vi "Dashboard Main.vi"() -> ()   [LabVIEW 2013]
uses:
  2014 Target Detection/TargetType.ctl
  <vilib>/event_ctls.llb/eventvkey.ctl
  <vilib>/Rock Robotics/WPI/Dashboard/WPI_DashboardLogging Global.vi
  <vilib>/Utility/config.llb/Write Key (String).vi
  <vilib>/Utility/config.llb/Write Key (I32).vi
  <vilib>/Utility/config.llb/NI_LVConfig.lvlib
panel:
  out "Image Message":string="Timeout in Camera Communications"
  in  "Rec Mode":enum32{"Stop", "Record", "Playback"}(radio)
  in  "Dashboard Tab":T1(tab)=enum."Auto"
  in  "Camera Settings":T2={"Frame Rate"=30, "Compression"=30, "Size"=1} {"Frame Rate" scale=1.0..30.0; "Size" items=["640x480", "320x240", "160x120"]}
  out "MotorSliders R":cluster{"MotorSlide1":dbl, "MotorSlide2":dbl}={"MotorSlide1"=0.0, "MotorSlide2"=-6.200012400024799e-05} {"MotorSlide2" scale=-1.0..1.0 scale format="%#_2e"; "MotorSlide1" scale=-1.0..1.0 scale format="%#_2e"}
  out "MotorChart R":cluster{"Numeric":dbl, "Numeric":dbl}(graph)={"Numeric"=0.0, "Numeric"=-6.200012400024799e-05}
  out "MotorSliders L":T3={"MotorSlide1"=0.0, "MotorSlide2"=-6.200012400024799e-05, "MotorSlide4 2"=12.519999504089355} {"MotorSlide4 2" scale=0.0..14.0 scale format="%#_2e"; "MotorSlide2" scale=-1.0..1.0 scale format="%#_2e"; "MotorSlide1" scale=-1.0..1.0 scale format="%#_2e"}
  out "MotorChart L":T4(graph)={"Numeric"=0.0, "Numeric"=-6.200012400024799e-05, "Battery"=12.5199995}
  out "JS1 Z":dbl(slide)=-1.0 scale=-1.0..1.0 scale format="%#_2e"
  out "Joystick 1":cluster{"X":dbl, "Y":dbl}[](graph)=[{"X"=-0.007874015748031496, "Y"=0.0}]
  out "JS Buttons 1":T5
  out "JS2 Z":dbl(slide) scale=-1.0..1.0 scale format="%#_2e"
  out "Joystick 2":cluster{"X":dbl, "Y":dbl}[](graph)
  out "JS Buttons 2":T5
  out "Mode":T6(ring)
  out "Camera IP":string="10.43.81.11"
  in  "DB Camera Config":bool
  out "fps":dbl=32.432432432432435 format="%#.1g"
  out "Mbps":dbl=3.953641040546432 format="%#.1g"
  out "Mbps 2":bool
  out "LED 1":bool
  in  "Slider 1":dbl(slide) scale=0.0..100.0
  out "Distances":T8(array[cluster])=[{"Distance (ft)"=9.467013752624329, "Target Center (-1 to 1)"={"X"=0.2125, "Y"=-0.19583333333333333}, "Left"=FALSE, "State"=enum."Hot"}]
  in  "Color Components":T9={"Hue"={96.67088317871094, 128.67088317871094}, "Sat"={183.00372314453125, 255.0}, "Val"={112.86207389831543, 166.60627937316895}} {"Val" scale=0.0..255.0; "Sat" scale=0.0..255.0; "Hue" scale=0.0..255.0 scale format="%#_3g"}
  in  "Checkbox 2":bool
  in  "Checkbox 1":bool
  in  "Test Slider":dbl(slide) scale=0.0..100.0 scale format="%#_3g"
  in  "On/Off":bool caption="Solenoid"
  in  "Test Name":u16(ring) items=["Select the test to run...", "Example Test", "-------------------------------", "List of tests is built in robot code.", "Replace with your own automated tests."]
  in  "Test Tree":string(tree)
  in  "Motor":cluster{"Value":dbl, "Enable":bool} {"Value" scale=-1.0..1.0 scale format="%#_3g"}
  out "Progress":T10 {"Test Progress" scale=0.0..100.0}
  in  "Rev/Fwd":cluster{"Forward":bool, "Reverse":bool}
  in  "Test Ring":u16(ring) items=["Auto", "Fixed indoor", "Fixed outdoor 1", "Fixed outdoor 2", "Fixed fluorescent 1", "Fixed fluorescent 2", "Hold current"]
  in  "Listbox":i32(listbox)
  out "Tree":string(tree)
  out "Camera Image":T11(plugin-control)
  in  "Enable":bool=TRUE
  # "Left"
  # "Front"
  # "Right"
  # "Battery"
  # "Customize by placing controls and indicators here and name to\nmatch Dashboard Variables on robot."
  # "This tab is a great place for autonomous settings and validation.\nCustomize by placing controls and indicators here and name to\nmatch Dashboard Variables on robot."
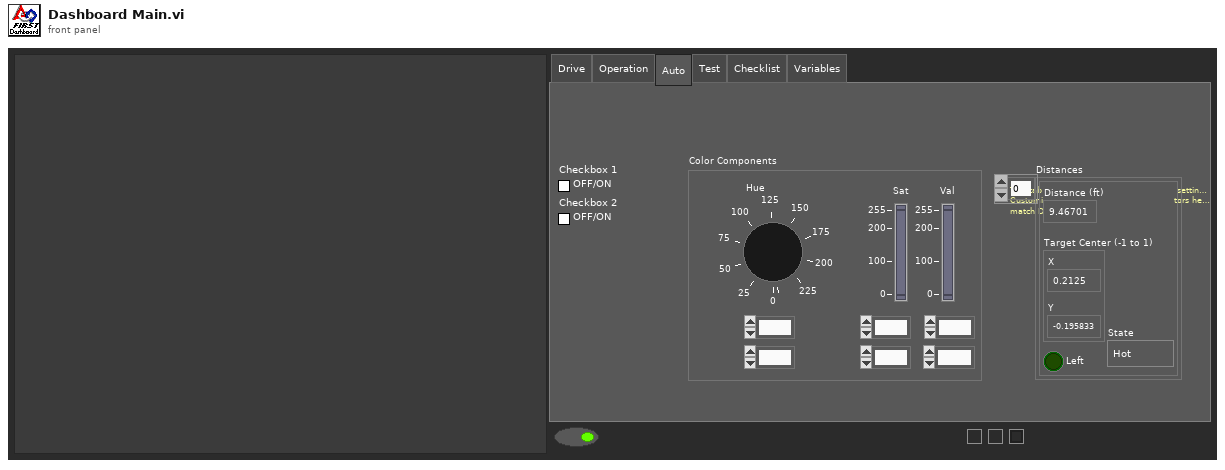
[diagram p1: front panel]
types:
  T1 = enum32{"Drive", "Operation", "Auto", "Test", "Checklist", "Variables"}
  T2 = cluster{"Frame Rate":i32, "Compression":i32, "Size":u16}
  T3 = cluster{"MotorSlide1":dbl, "MotorSlide2":dbl, "MotorSlide4 2":dbl}
  T4 = cluster{"Numeric":dbl, "Numeric":dbl, "Battery":sgl}
  T5 = cluster{bool, bool, bool, bool, bool, bool, bool, bool, bool, bool, bool, bool}
  T6 = enum8{"Tele-Op Disabled", "Tele-Op Enabled", "Auto Disabled", "Auto Enabled", "Test Disabled", "Test Enabled", ""}
  T7 = typedef "TargetType.ctl" = enum16{"Not Hot", "Hot"}
  T8 = cluster{"Distance (ft)":dbl, "Target Center (-1 to 1)":cluster{"X":dbl, "Y":dbl}, "Left":bool, "State":T7}[]
  T9 = cluster{"Hue":cluster{dbl, dbl}, "Sat":cluster{dbl, dbl}, "Val":cluster{dbl, dbl}}
  T10 = cluster{"Test Progress":u8, "Test Progress Text":string}
  T11 = typedef "IMAQ Image.ctl" = refnum<image>
  T12 = typedef "Image Type" = u32
  T13 = cluster{cluster{dbl, dbl}, cluster{dbl, dbl}, cluster{dbl, dbl}}
  T14 = cluster{"Digital Inputs":bool[], "Digital Outputs":bool[]}
  T15 = cluster{"Competition mode":bool, "Robot Link":bool, "Autonomous":bool, "Enabled":bool, "E-Stop":bool, "Simulated":bool, "TestMode":bool, "Docked Window":bool}
  T16 = cluster{"Boolean Array[0]":bool, "Boolean Array[1]":bool, "Boolean Array[2]":bool, "Boolean Array[3]":bool, "Boolean Array[4]":bool, "Boolean Array[5]":bool, "Boolean Array[6]":bool, "Boolean Array[7]":bool, "Boolean Array[8]":bool, "Boolean Array[9]":bool, "Boolean Array[10]":bool, "Boolean Array[11]":bool}
  T17 = typedef "NI_LVConfig.lvlib/Config Data RefNum.ctl" = refnum<k1>
  T18 = typedef "eventvkey.ctl" = enum16{"ASCII", "Enter", "Return", "Shift", "Ctrl", "Alt", "Cmd", "Opt", "Caps", "NumLock", "Clear", "Break", "Up", "Down", "Left", "Right", "Insert", "Delete", "Home", "End", "PageUp", "PageDown", "Escape", "Help", "Pause", "ScrollLock", "F1", "F2", "F3", "F4", "F5", "F6", "F7", "F8", "F9", "F10", "F11", "F12", "F13", "F14", "F15", "F16", "F17", "F18", "F19", "F20", "F21", "F22", "F23", "F24", "Play", "VolumeUp", "VolumeDown", "Mute", "Two Byte Char"}
  T19 = cluster{"Image Size":bool, "Image Type":bool, "Pixel Value":bool, "ROI Information":bool, "Zoom Factor":bool}
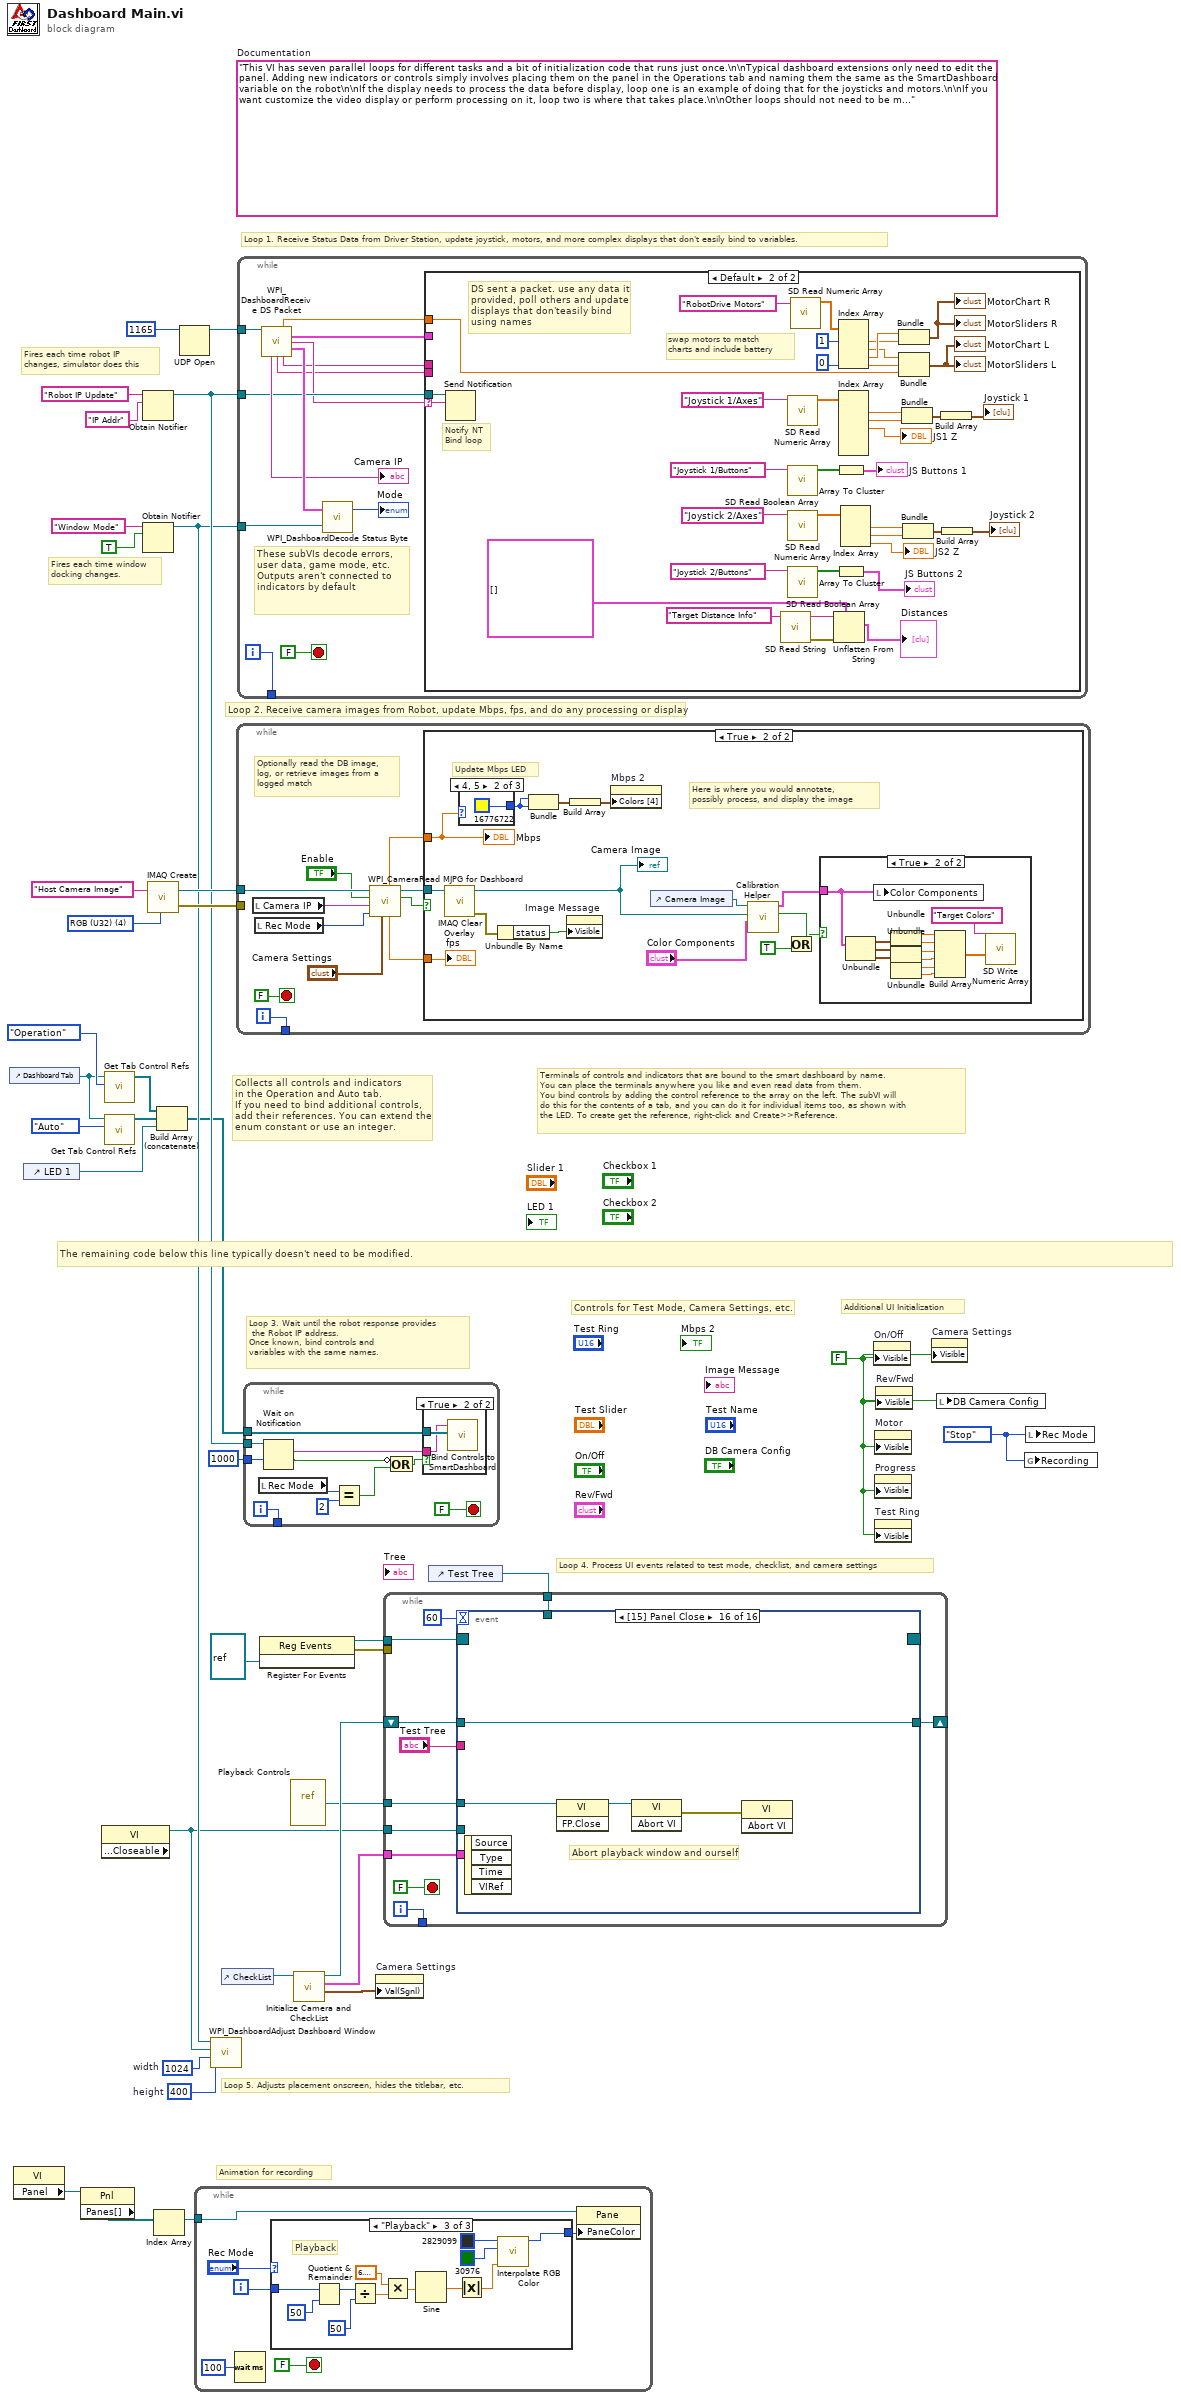
[diagram p0: block diagram]
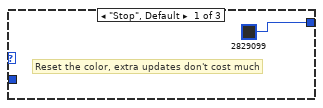
[diagram p2: hidden frame]
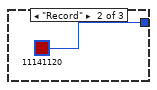
[diagram p3: hidden frame]
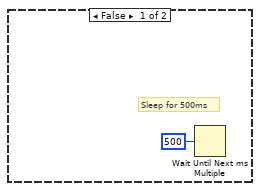
[diagram p5: hidden frame]
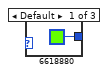
[diagram p7: hidden frame]
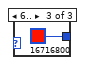
[diagram p8: hidden frame]
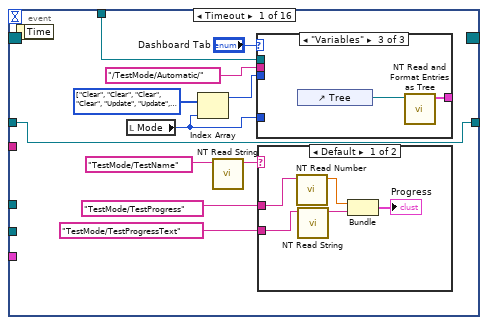
[diagram p9: hidden frame]
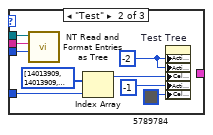
[diagram p11: hidden frame]
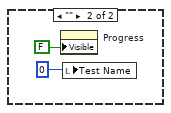
[diagram p12: hidden frame]
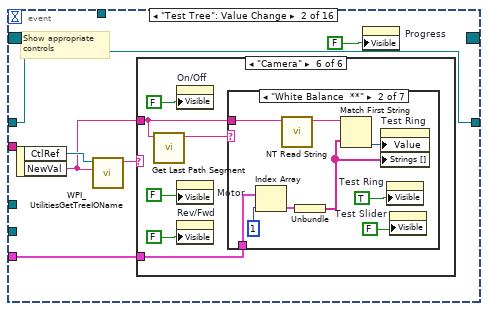
[diagram p13: hidden frame]
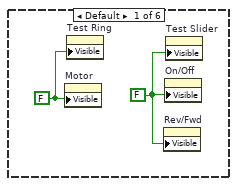
[diagram p14: hidden frame]
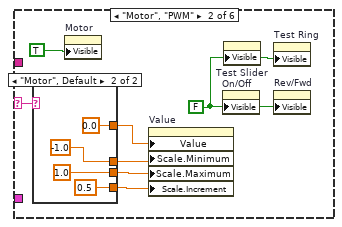
[diagram p15: hidden frame]
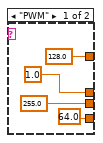
[diagram p16: hidden frame]
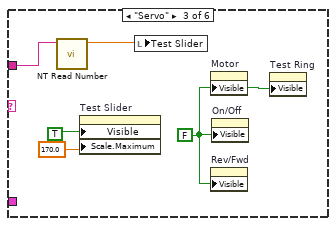
[diagram p17: hidden frame]
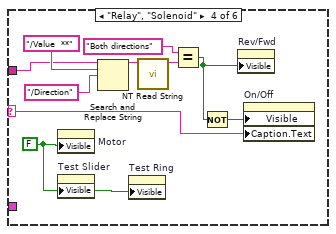
[diagram p18: hidden frame]
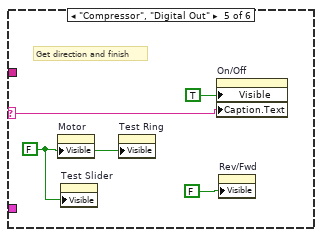
[diagram p19: hidden frame]
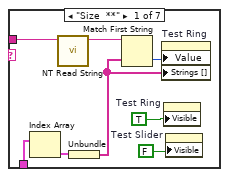
[diagram p20: hidden frame]
diagram:
  w8 = enum32{"Stop", "Record", "Playback"}."Stop" ("Rec Mode")
  w11 = 400  # height
  w12 = 1024  # width
  w25 = FALSE ("Visible")
  (unwired) "This VI has seven parallel loops for different tasks and a bit of initialization code that runs just once.\n\nTypical dashboard extensions only need to edit the panel. Adding new indicators or controls simply involves placing them on the panel in the Operations tab and naming them the same as the SmartDashboard variable on the robot\n\nIf the display needs to process the data before display, loop one is an example of doing that for the joysticks and motors.\n\nIf you want customize the video display or perform processing on it, loop two is where that takes place.\n\nOther loops should not need to be modified. They are pretty standard, and document the task they perform."  # Documentation
  w35 = T12 4 items=["Grayscale (U8)", "Grayscale (I16)", "Grayscale (SGL)", "Complex (CSG)", "RGB (U32)", "HSL (U32)", "RGB (U64)"] ("Image Type")
  # "Controls for Test Mode, Camera Settings, etc."
  # "Additional UI Initialization"
  # "Animation for recording"
  # "Fires each time robot IP\nchanges, simulator does this"
  # "Fires each time window\ndocking changes."
  # "Collects all controls and indicators\nin the Operation and Auto tab.\nIf you need to bind additional controls,\nadd their references. You can extend the\nenum constant or use an integer."
  # "The remaining code below this line typically doesn't need to be modified."
  # "Loop 4. Process UI events related to test mode, checklist, and camera settings"
  # "Terminals of controls and indicators that are bound to the smart dashboard by name.\nYou can place the terminals anywhere you like and even read data from them.\nYou bind controls by adding the control reference to the array on the left. The subVI will\ndo this for the contents of a tab, and you can do it for individual items too, as shown with\nthe LED. To create get the reference, right-click and Create>>Reference."
  # "Loop 3. Wait until the robot response provides\n the Robot IP address.\nOnce known, bind controls and\nvariables with the same names."
  # "Loop 5. Adjusts placement onscreen, hides the titlebar, etc."
  # "Loop 1. Receive Status Data from Driver Station, update joystick, motors, and more complex displays that don't easily bind to variables."
  # "Loop 2. Receive camera images from Robot, update Mbps, fps, and do any processing or display"
  n1 = control-ref of="Dashboard Tab"() -> (w6:refnum<vi>)
  n2 = property class="VI"() -> ("Panel"=w19:refnum<vi>)  [unwired: 2 in, 2 out]
  n3 = control-ref of="LED 1"() -> (w1:refnum<vi>)
  n4 = property class="Pnl"(reference=w19) -> ("Panes[]"=w20:refnum<vi>[])  [unwired: 1 in, 2 out]
  n5 = property class="VI" props=["Front Panel.Closeable"]() -> (reference out=w7:refnum<vi>)  [unwired: 2 in, 2 out]
  n6 = call <vilib>:"Get Tab Control Refs.vi"("Page Index"=T1."Operation" ("Dashboard Tab"), "TabControl in"=w6) -> ("ControlsOnPage"=w4:refnum<vi>[])  [unwired: 9 in]
  n7 = call <vilib>:"Get Tab Control Refs.vi"("Page Index"=T1."Auto" ("Dashboard Tab"), "TabControl in"=w6) -> ("ControlsOnPage"=w5:refnum<vi>[])  [unwired: 9 in]
  n8 = Obtain Notifier(name (unnamed)="Robot IP Update", notification data type="IP Addr" ("name (unnamed)")) -> (notifier out=w29:refnum<notifier>)  [unwired: 2 in, 2 out]
  n9 = Obtain Notifier(name (unnamed)="Window Mode", notification data type=TRUE) -> (notifier out=w10:refnum<notifier>)  [unwired: 2 in, 2 out]
  n10 = call "IMAQ Create"("Image Name"="Host Camera Image", "Image Type"=w35) -> ("New Image"=w33:T11, "error out"=w32:errorcluster)  [unwired: 2 in, 1 out]
  n11 = Index Array(array=w20) -> (element=w18:refnum<vi>)  [unwired: 1 in]
  n12 = Build Array (concatenate)(w4, w5, w1) -> (w3:refnum<vi>[])
  n13 = UDP Open(11:u16 1165 ("port")) -> (port=w36:refnum<k16>)  [unwired: 2 in, 4 out]
  n14 = while {
    tunnel: w18 -> [w39]
    i -> [w42]
    stop <- FALSE stop-if-true
    n15 = Wait (ms)(milliseconds to wait=u32 100) -> ()  [unwired: 1 out]
    n16 = case shown="\"Playback\"" "Rec Mode" {
      tunnel: w42 -> [_ _ w57]
      tunnel: [u32 2829099 ("Base Color") u32 11141120 ("Target Color") w46] -> w38
      frame "Stop", Default {
        # "Reset the color, extra updates don't cost much"
      }
      frame "Record" {
      }
      frame "Playback" {
        # "Playback"
        n17 = Quotient & Remainder(x=w57, y=u32 50 ("milliseconds to wait")) -> (x-y*floor(x/y)=w53:u32)  [unwired: 1 out]
        n18 = Divide(x=w53, y=u32 50 ("milliseconds to wait")) -> (x/y=w50:dbl)
        n19 = Multiply(x=6.283185307179586, y=w50) -> (x*y=w55:dbl)
        n20 = Sine(x=w55) -> (sin(x)=w54:dbl)
        n21 = Absolute Value(x=w54) -> (abs(x)=w47:dbl)
        n22 = call "Interpolate RGB Color.vi"("Proportion"=w47, "Target Color"=u32 30976, "Base Color"=u32 2829099) -> ("Result Color"=w46:u32)  [unwired: 8 in]
      }
    }
    n23 = property class="Pane"(reference=w39, "PaneColor"=w38) -> ()  [unwired: 1 in, 2 out]
  }
  n24 = call <vilib>:"WPI_DashboardAdjust Dashboard Window.vi"("height"=w11, "width"=w12, "reference in"=w7, "Notifier in"=w10) -> ()  [unwired: 8 in]
  n25 = control-ref of="CheckList"() -> (w9:refnum<vi>)
  n26 = while {
    tunnel: w33 -> [w66]
    tunnel: w32 -> [_]
    tunnel: [w67] -> _
    i -> [w67]
    stop <- FALSE stop-if-true
    # "Optionally read the DB image,\nlog, or retrieve images from a\nlogged match"
    n27 = local read "Camera IP"() -> (w59:string)
    n28 = local read "Rec Mode"() -> (w58:enum32{"Stop", "Record", "Playback"})
    n29 = call <vilib>:"WPI_CameraRead MJPG for Dashboard.vi"("Camera Settings"="Camera Settings", "Rec Mode"=w58, "Camera IP"=w59, "Enable"="Enable", "Refnum in"=w66) -> ("Active"=w63:bool, "Refnum out"=w65:T11, "FPS"=w62:dbl, "Bandwidth (Mbps)"=w61:dbl)  [unwired: 3 in]
    n30 = case shown="True" w63 {
      tunnel: w65 -> [_ w79]
      tunnel: w61 -> [_ w78]
      tunnel: w62 -> [_ w77]
      frame False {
        # "Sleep for 500ms"
        n31 = Wait Until Next ms Multiple(millisecond multiple=u32 500) -> ()  [unwired: 1 out]
      }
      frame True {
        # "Here is where you would annotate,\npossibly process, and display the image"
        # "Update Mbps LED"
        n32 = call "IMAQ Clear Overlay"("Image"=w79) -> ("error out"=w83:errorcluster, "Image Out"=w76:T11)  [unwired: 2 in, 7 out]
        "Camera Image" <- w76
        n33 = case shown="4, 5" w78 {
          tunnel: [u32 6618880 ("Color Box") u32 16776722 ("Color Box") u32 16716800 ("Color Box")] -> w80
          frame Default {
          }
          frame 4, 5 {
          }
          frame 6.. {
          }
        }
        n34 = Unbundle By Name(w83) -> ("status"=w84:bool)
        n35 = Bundle("Color Box"=w80, "Color Box"=w80) -> (w82:cluster{"Color Box":u32, "Color Box":u32})  [unwired: 1 out]
        n36 = property on="Image Message" class="Str"("Visible"=w84) -> ()  [unwired: 2 in, 2 out]
        n37 = Build Array(w82) -> (w81:cluster{"Color Box":u32, "Color Box":u32}[])
        n38 = property on="Mbps 2" class="Bool (strict)"("Colors [4]"=w81) -> ()  [unwired: 2 in, 2 out]
        n39 = control-ref of="Camera Image"() -> (w75:refnum<vi>)
        n40 = call "Calibration Helper.vi"("Color Components"="Color Components", "Image"=w76, "Image Ctl Refnum"=w75) -> ("Changed"=w72:bool, "output color"=w73:T13)  [unwired: 7 in]
        n41 = Or(x=w72, y=TRUE) -> (x .or. y?=w70:bool)
        n42 = case shown="True" w70 {
          tunnel: w73 -> [_ w96]
          frame False {
          }
          frame True {
            n43 = Unbundle(w96) -> (w95:cluster{dbl, dbl}, w94:cluster{dbl, dbl}, w93:cluster{dbl, dbl})
            n44 = local write "Color Components"(w96) -> ()
            n45 = Unbundle(w95) -> (w92:dbl, w91:dbl)
            n46 = Unbundle(w94) -> (w90:dbl, w89:dbl)
            n47 = Unbundle(w93) -> (w88:dbl, w87:dbl)
            n48 = Build Array(w92, w91, w90, w89, w88, w87) -> (w86:dbl[])
            n49 = call <vilib>:"SD Write Numeric Array.vi"("Numeric Array"=w86, "Name"="Target Colors") -> ()  [unwired: 8 in, 2 out]
          }
        }
        "Mbps" <- w78
        "fps" <- w77
      }
    }
  }
  n50 = while {
    tunnel: w36 -> [w110]
    tunnel: w29 -> [w105]
    tunnel: w10 -> [w109]
    tunnel: [w106] -> _
    i -> [w106]
    stop <- FALSE stop-if-true
    # "These subVIs decode errors, user data, game mode, etc.\nOutputs aren't connected to indicators by default"
    n51 = call <vilib>:"WPI_DashboardReceive DS Packet.vi"("Recv Socket"=w110) -> ("Battery"=w100:sgl, "Driver Station"=w101:T14, "Robot IP Address"=w104:string, "Status"=w111:T15, "Camera IP Address"=→"Camera IP":string, "Low Priority User Data"=w103:string, "High Priority User Data"=w102:string)  [unwired: 1 in, 7 out]
    n52 = call <vilib>:"WPI_DashboardDecode Status Byte.vi"("Window Mode Notifier"=w109, "Status"=w111) -> ("Mode"=→"Mode":T6)  [unwired: 1 out]
    n53 = case shown="Default" w104 {
      selector: w104 -> [_ w128]
      tunnel: w105 -> [_ w129]
      tunnel: w103 -> [_ _]
      tunnel: w102 -> [_ _]
      tunnel: w101 -> [_ _]
      tunnel: w100 -> [_ w127]
      frame "0.0.0.0" {
        # "DS not sending packets, or no robot exists yet.\nDon't poll the variables"
      }
      frame Default {
        # "Notify NT\nBind loop"
        # "DS sent a packet. use any data it\nprovided, poll others and update\ndisplays that don'teasily bind\nusing names"
        # "swap motors to match\ncharts and include battery"
        n54 = Send Notification(notification=w128, notifier=w129) -> ()  [unwired: 1 in, 2 out]
        n55 = call <vilib>:"SD Read String.vi"("Name"="Target Distance Info") -> ("error out"=w117:errorcluster, "String"=w116:string)  [unwired: 8 in, 1 out]
        n56 = call <vilib>:"SD Read Numeric Array.vi"("Name"="Joystick 1/Axes") -> ("Numeric Array"=w145:dbl[])  [unwired: 8 in, 2 out]
        n57 = call <vilib>:"SD Read Boolean Array.vi"("Name"="Joystick 1/Buttons") -> ("Boolean Array"=w147:bool[])  [unwired: 8 in, 2 out]
        n58 = call <vilib>:"SD Read Numeric Array.vi"("Name"="Joystick 2/Axes") -> ("Numeric Array"=w139:dbl[])  [unwired: 8 in, 2 out]
        n59 = call <vilib>:"SD Read Boolean Array.vi"("Name"="Joystick 2/Buttons") -> ("Boolean Array"=w138:bool[])  [unwired: 8 in, 2 out]
        n60 = call <vilib>:"SD Read Numeric Array.vi"("Name"="RobotDrive Motors") -> ("Numeric Array"=w126:dbl[])  [unwired: 8 in, 2 out]
        n61 = Unflatten From String(type=T8 [] ("Distances"), binary string=w116, error in (no error)=w117) -> (value=→"Distances":T8)  [unwired: 2 in, 2 out]
        n62 = Array To Cluster(array=w147) -> (cluster=→"JS Buttons 1":T16)
        n63 = Array To Cluster(array=w138) -> (cluster=→"JS Buttons 2":T16)
        n64 = Index Array(array=w126, index #1=1, index #4=0) -> (element #1=w122:dbl, element #2=w121:dbl, element #3=w123:dbl, element #4=w118:dbl)  [unwired: 2 in]
        n65 = Index Array(array=w145) -> (element #1=w142:dbl, element #2=w143:dbl, element #3=→"JS1 Z":dbl)  [unwired: 6 in, 3 out]
        n66 = Index Array(array=w139) -> (element #1=w134:dbl, element #2=w133:dbl, element #3=→"JS2 Z":dbl)  [unwired: 3 in]
        n67 = Bundle("Numeric"=w123, "Numeric"=w122) -> (→"MotorChart R" →"MotorSliders R":cluster{"Numeric":dbl, "Numeric":dbl})  [unwired: 1 in]
        n68 = Bundle("Numeric"=w121, "Numeric"=w118, "Battery"=w127) -> (→"MotorChart L" →"MotorSliders L":T4)  [unwired: 1 in]
        n69 = Bundle("Numeric"=w142, "Numeric"=w143) -> (w141:cluster{"Numeric":dbl, "Numeric":dbl})  [unwired: 1 in]
        n70 = Bundle("Numeric"=w134, "Numeric"=w133) -> (w135:cluster{"Numeric":dbl, "Numeric":dbl})  [unwired: 1 in]
        n71 = Build Array(w141) -> (→"Joystick 1":cluster{"Numeric":dbl, "Numeric":dbl}[])
        n72 = Build Array(w135) -> (→"Joystick 2":cluster{"Numeric":dbl, "Numeric":dbl}[])
      }
    }
  }
  n73 = while {
    tunnel: w3 -> [w161]
    tunnel: w29 -> [w159]
    tunnel: [w157] -> _
    tunnel: u32 1000 ("milliseconds to wait") -> [w156]
    i -> [w157]
    stop <- FALSE stop-if-true
    n74 = local read "Rec Mode"() -> (w152:enum32{"Stop", "Record", "Playback"})
    n75 = Wait on Notification(notifier=w159, timeout in ms (-1)=w156) -> (notification=w158:string, timed out?=w154:bool)  [unwired: 2 in, 2 out]
    n76 = Equal?(x=w152, y=u16 2 ("Rec Mode")) -> (x = y?=w153:bool)
    n77 = Compound Arithmetic op=OR(invert w154, w153) -> (w155:bool)
    n78 = case shown="True" w155 {
      tunnel: w161 -> [_ w163]
      tunnel: w158 -> [_ w162]
      frame False {
      }
      frame True {
        n79 = call <vilib>:"Bind Controls to SmartDashboard.vi"("Bound Control Refs"=w163, "Server IP Address"=w162) -> ()  [unwired: 10 in]
      }
    }
  }
  n80 = register-events(refnum<vi> refnum) -> (reference out=w16:refnum<event-registration>, error out=w15:errorcluster)  [unwired: 2 in]
  n81 = vi-ref "Playback Controls.vi"() -> (w17:refnum<vi>)
  n82 = call "Initialize Camera and CheckList.vi"("ListBox in"=w9) -> ("Cluster"=w23:cluster{"value":i32, "value":i32, "index":i32}, "Array"=w24:cluster{string[]}[], "File Refnum"=w22:T17)  [unwired: 8 in]
  n83 = property on="Camera Settings" class="Clust (strict)"("Val(Sgnl)"=w23) -> ()  [unwired: 2 in, 2 out]
  n84 = control-ref of="Test Tree"() -> (w21:refnum<vi>)
  n85 = while {
    tunnel: w24 -> [w171]
    shift-right: [w170] -> _
    shift-left: w22 -> [w169]
    tunnel: [w168] -> _
    tunnel: w21 -> [w167]
    tunnel: w17 -> [w166]
    tunnel: w16 -> [w165]
    tunnel: w15 -> [_]
    tunnel: w7 -> [w164]
    i -> [w168]
    stop <- FALSE stop-if-true
    n86 = event shown="[15] Panel Close" {
      selector: w165 -> [_ _ _ _ _ _ _ _ _ _ _ _ _ _ _ _]
      dyn-events: [_ _ _ _ _ _ _ _ _ _ _ _ _ w409 _ _] -> _
      timeout: u32 60 ("milliseconds to wait") -> [_ _ _ _ _ _ _ _ _ _ _ _ _ _ _ _]
      tunnel: w167 -> [w181 _ _ _ _ _ _ _ _ _ _ _ _ _ _ _]
      tunnel: "Test Tree" -> [_ _ _ _ _ _ _ _ w378 w386 w388 w392 w400 _ _ _]
      tunnel: w171 -> [_ w205 _ _ _ _ w342 w372 _ _ _ _ _ _ _ _]
      tunnel: [w175 w204 w303 w308 w316 w328 w341 w365 w377 w384 w387 w391 w399 w411 w425 w426] -> w170
      tunnel: w169 -> [w175 w204 w303 w308 w316 w328 w340 w365 w377 w384 w387 w391 w399 w411 w425 w426]
      tunnel: w166 -> [_ _ _ _ _ _ _ _ _ _ _ _ _ w412 _ w429]
      tunnel: w164 -> [_ _ _ _ _ _ _ _ _ _ _ _ _ w407 _ _]
      event Timeout {
        w180 = enum16{"Update", "Clear"}[] [enum."Clear", enum."Clear", enum."Clear", enum."Clear", enum."Update", enum."Update", enum."Clear"] items=["Update", "Clear"]
        n87 = event-data() -> ()  [unwired: 1 in, 1 out]
        n88 = local read "Mode"() -> (w178:T6)
        n89 = Index Array(array=w180, index=w178) -> (element=w179:enum16{"Update", "Clear"})
        n90 = call <vilib>:"NT Read String.vi"("Name"="TestMode/TestName") -> ("String"=w184:string)  [unwired: 9 in, 1 out]
        n91 = case shown="\"Variables\"" "Dashboard Tab" {
          tunnel: w181 -> [_ w194 _]
          tunnel: "/TestMode/Automatic/" ("Name Pattern") -> [_ w193 _]
          tunnel: w179 -> [_ w192 _]
          tunnel: w178 -> [_ w190 _]
          tunnel: [_ _ w196] -> _
          frame "Operation", Default {
          }
          frame "Test" {
            w189 = -2 ("Active Item:Row Number")
            n92 = call <vilib>:"NT Read and Format Entries as Tree.vi"("Operation"=w192, "Name Pattern"=w193, "Tree Refnum"=w194) -> ()  [unwired: 7 in, 2 out]
            n93 = Index Array(array=u32[] [14013909, 14013909, 14013909, 14013909, 14013909, 16777215, 14013909], index=w190) -> (element=w188:u32)
            n94 = property on="Test Tree" class="Tree (strict)"("Active Item Row Number"=w189, "ActiveColNum"=w189, "CellBG"=w188, "Active Item Row Number"=-1 ("Active Item:Row Number"), "CellBG"=u32 5789784 ("Color Box")) -> ()  [unwired: 2 in, 2 out]
          }
          frame "Variables" {
            n95 = control-ref of="Tree"() -> (w195:refnum<vi>)
            n96 = call <vilib>:"NT Read and Format Entries as Tree.vi"("Tree Refnum"=w195) -> ("Formatted Strings"=w196:cluster{"Name":string, "Value":string}[])  [unwired: 9 in, 1 out]
          }
        }
        n97 = case shown="Default" w184 {
          tunnel: "TestMode/TestProgress" ("Name") -> [w198 _]
          tunnel: "TestMode/TestProgressText" ("Name") -> [w197 _]
          frame Default {
            n98 = call <vilib>:"NT Read Number.vi"("Name"=w198) -> ("Numeric"=w199:dbl)  [unwired: 9 in, 1 out]
            n99 = call <vilib>:"NT Read String.vi"("Name"=w197) -> ("String"=w200:string)  [unwired: 9 in, 1 out]
            n100 = Bundle("Numeric"=w199, "String"=w200) -> (→"Progress":cluster{"Numeric":dbl, "String":string})  [unwired: 1 in]
          }
          frame "" {
            n101 = property on="Progress" class="Clust (strict)"("Visible"=FALSE) -> ()  [unwired: 2 in, 2 out]
            n102 = local write "Test Name"(u16 0) -> ()
          }
        }
      }
      event "Test Tree": Value Change {
        # "Show appropriate\ncontrols"
        n103 = event-data() -> ("CtlRef"=w208:refnum<vi>, "NewVal"=w206:string)  [unwired: 1 in]
        n104 = call <vilib>:"WPI_UtilitiesGetTreeIOName.vi"("NewVal"=w206, "TreeControl in"=w208) -> ("I/O Name"=w209:string)  [unwired: 9 in]
        n105 = case shown="\"Camera\"" w209 {
          selector: w209 -> [_ w216 _ w234 w243 _]
          tunnel: w206 -> [_ _ w231 w233 _ w250]
          tunnel: w205 -> [_ _ _ _ _ w249]
          frame Default {
            w211 = FALSE ("Visible")
            w210 = FALSE ("Visible")
            n106 = property on="Motor" class="Clust (strict)"("Visible"=w210) -> ()  [unwired: 2 in, 2 out]
            n107 = property on="Test Ring" class="Ring (strict)"("Visible"=w210) -> ()  [unwired: 2 in, 2 out]
            n108 = property on="Rev/Fwd" class="Clust (strict)"("Visible"=w211) -> ()  [unwired: 2 in, 2 out]
            n109 = property on="On/Off" class="Bool (strict)"("Visible"=w211) -> ()  [unwired: 2 in, 2 out]
            n110 = property on="Test Slider" class="Slide (strict)"("Visible"=w211) -> ()  [unwired: 2 in, 2 out]
          }
          frame "Motor", "PWM" {
            w217 = FALSE ("Visible")
            n111 = case shown="\"Motor\", Default" w216 {
              tunnel: [1.0 ("Value") -1.0 ("Value")] -> w215
              tunnel: [255.0 ("Value") 1.0 ("Value")] -> w214
              tunnel: [128.0 ("Value") 0.0 ("Value")] -> w213
              tunnel: [64.0 ("Value") 0.5 ("Value")] -> w212
              frame "PWM" {
              }
              frame "Motor", Default {
              }
            }
            n112 = property on="Motor" class="Clust (strict)"("Visible"=TRUE) -> ()  [unwired: 2 in, 2 out]
            n113 = property on="Value" class="Slide (strict)"("Value"=w213, "Scale.Minimum"=w215, "Scale.Maximum"=w214, "Scale.Increment"=w212) -> ()  [unwired: 2 in, 2 out]
            n114 = property on="On/Off" class="Bool (strict)"("Visible"=w217) -> ()  [unwired: 2 in, 2 out]
            n115 = property on="Test Slider" class="Slide (strict)"("Visible"=w217) -> ()  [unwired: 2 in, 2 out]
            n116 = property on="Test Ring" class="Ring (strict)"("Visible"=w217) -> ()  [unwired: 2 in, 2 out]
            n117 = property on="Rev/Fwd" class="Clust (strict)"("Visible"=w217) -> ()  [unwired: 2 in, 2 out]
          }
          frame "Servo" {
            w229 = FALSE ("Visible")
            n118 = call <vilib>:"NT Read Number.vi"("Name"=w231) -> ("Numeric"=w230:dbl)  [unwired: 9 in, 1 out]
            n119 = property on="Test Slider" class="Slide (strict)"("Visible"=TRUE, "Scale.Maximum"=170.0 ("Scale.Range:Maximum")) -> ()  [unwired: 2 in, 2 out]
            n120 = local write "Test Slider"(w230) -> ()
            n121 = property on="Motor" class="Clust (strict)"("Visible"=w229) -> ()  [unwired: 2 in, 2 out]
            n122 = property on="Rev/Fwd" class="Clust (strict)"("Visible"=w229) -> ()  [unwired: 2 in, 2 out]
            n123 = property on="On/Off" class="Bool (strict)"("Visible"=w229) -> ()  [unwired: 2 in, 2 out]
            n124 = property on="Test Ring" class="Ring (strict)"("Visible"=w229) -> ()  [unwired: 2 in, 2 out]
          }
          frame "Relay", "Solenoid" {
            w232 = FALSE ("Visible")
            n125 = property on="Motor" class="Clust (strict)"("Visible"=w232) -> ()  [unwired: 2 in, 2 out]
            n126 = property on="Test Slider" class="Slide (strict)"("Visible"=w232) -> ()  [unwired: 2 in, 2 out]
            n127 = Search and Replace String(input string=w233, search string="/Value  **", replace string="/Direction") -> (result string=w239:string)  [unwired: 5 in, 3 out]
            n128 = property on="Test Ring" class="Ring (strict)"("Visible"=w232) -> ()  [unwired: 2 in, 2 out]
            n129 = call <vilib>:"NT Read String.vi"("Name"=w239) -> ("String"=w237:string)  [unwired: 9 in, 1 out]
            n130 = Equal?(x="Both directions", y=w237) -> (x = y?=w235:bool)
            n131 = Not(x=w235) -> (.not. x?=w236:bool)
            n132 = property on="Rev/Fwd" class="Clust (strict)"("Visible"=w235) -> ()  [unwired: 2 in, 2 out]
            n133 = property on="On/Off" class="Bool (strict)"("Visible"=w236, "Caption.Text"=w234) -> ()  [unwired: 2 in, 2 out]
          }
          frame "Compressor", "Digital Out" {
            w242 = FALSE ("Visible")
            # "Get direction and finish"
            n134 = property on="Motor" class="Clust (strict)"("Visible"=w242) -> ()  [unwired: 2 in, 2 out]
            n135 = property on="Test Slider" class="Slide (strict)"("Visible"=w242) -> ()  [unwired: 2 in, 2 out]
            n136 = property on="Test Ring" class="Ring (strict)"("Visible"=w242) -> ()  [unwired: 2 in, 2 out]
            n137 = property on="On/Off" class="Bool (strict)"("Visible"=TRUE, "Caption.Text"=w243) -> ()  [unwired: 2 in, 2 out]
            n138 = property on="Rev/Fwd" class="Clust (strict)"("Visible"=FALSE) -> ()  [unwired: 2 in, 2 out]
          }
          frame "Camera" {
            n139 = call <vilib>:"Get Last Path Segment.vi"("String in"=w250) -> ("String out"=w251:string)  [unwired: 10 in]
            n140 = property on="On/Off" class="Bool (strict)"("Visible"=FALSE) -> ()  [unwired: 2 in, 2 out]
            n141 = property on="Motor" class="Clust (strict)"("Visible"=FALSE) -> ()  [unwired: 2 in, 2 out]
            n142 = property on="Rev/Fwd" class="Clust (strict)"("Visible"=FALSE) -> ()  [unwired: 2 in, 2 out]
            n143 = case shown="\"White Balance  **\"" w251 {
              tunnel: w250 -> [w257 w266 w275 w284 w293 _ w299]
              tunnel: w249 -> [w255 w263 w272 w281 w290 _ _]
              frame "Size  **" {
                n144 = Index Array(array=w255) -> (element=w254:cluster{string[]})  [unwired: 1 in]
                n145 = call <vilib>:"NT Read String.vi"("Name"=w257) -> ("String"=w256:string)  [unwired: 9 in, 1 out]
                n146 = Unbundle(w254) -> (w252:string[])
                n147 = Match First String(2:w252, 3:w256) -> (0:w253:i32)  [unwired: 1 out]
                n148 = property on="Test Ring" class="Ring (strict)"("Value"=w253, "Strings []"=w252) -> ()  [unwired: 2 in, 2 out]
                n149 = property on="Test Ring" class="Ring (strict)"("Visible"=TRUE) -> ()  [unwired: 2 in, 2 out]
                n150 = property on="Test Slider" class="Slide (strict)"("Visible"=FALSE) -> ()  [unwired: 2 in, 2 out]
              }
              frame "White Balance  **" {
                n151 = Index Array(array=w263, index=1) -> (element=w264:cluster{string[]})
                n152 = call <vilib>:"NT Read String.vi"("Name"=w266) -> ("String"=w265:string)  [unwired: 9 in, 1 out]
                n153 = Unbundle(w264) -> (w261:string[])
                n154 = Match First String(2:w261, 3:w265) -> (0:w260:i32)  [unwired: 1 out]
                n155 = property on="Test Ring" class="Ring (strict)"("Value"=w260, "Strings []"=w261) -> ()  [unwired: 2 in, 2 out]
                n156 = property on="Test Ring" class="Ring (strict)"("Visible"=TRUE) -> ()  [unwired: 2 in, 2 out]
                n157 = property on="Test Slider" class="Slide (strict)"("Visible"=FALSE) -> ()  [unwired: 2 in, 2 out]
              }
              frame "Exposure  **" {
                n158 = Index Array(array=w272, index=2) -> (element=w273:cluster{string[]})
                n159 = call <vilib>:"NT Read String.vi"("Name"=w275) -> ("String"=w274:string)  [unwired: 9 in, 1 out]
                n160 = Unbundle(w273) -> (w269:string[])
                n161 = Match First String(2:w269, 3:w274) -> (0:w270:i32)  [unwired: 1 out]
                n162 = property on="Test Ring" class="Ring (strict)"("Value"=w270, "Strings []"=w269) -> ()  [unwired: 2 in, 2 out]
                n163 = property on="Test Ring" class="Ring (strict)"("Visible"=TRUE) -> ()  [unwired: 2 in, 2 out]
                n164 = property on="Test Slider" class="Slide (strict)"("Visible"=FALSE) -> ()  [unwired: 2 in, 2 out]
              }
              frame "Exposure Priority  **" {
                n165 = Index Array(array=w281, index=3) -> (element=w282:cluster{string[]})
                n166 = call <vilib>:"NT Read String.vi"("Name"=w284) -> ("String"=w283:string)  [unwired: 9 in, 1 out]
                n167 = Unbundle(w282) -> (w278:string[])
                n168 = Match First String(2:w278, 3:w283) -> (0:w279:i32)  [unwired: 1 out]
                n169 = property on="Test Ring" class="Ring (strict)"("Value"=w279, "Strings []"=w278) -> ()  [unwired: 2 in, 2 out]
                n170 = property on="Test Ring" class="Ring (strict)"("Visible"=TRUE) -> ()  [unwired: 2 in, 2 out]
                n171 = property on="Test Slider" class="Slide (strict)"("Visible"=FALSE) -> ()  [unwired: 2 in, 2 out]
              }
              frame "Color Enable  **" {
                n172 = Index Array(array=w290, index=4) -> (element=w291:cluster{string[]})
                n173 = call <vilib>:"NT Read String.vi"("Name"=w293) -> ("String"=w292:string)  [unwired: 9 in, 1 out]
                n174 = Unbundle(w291) -> (w287:string[])
                n175 = Match First String(2:w287, 3:w292) -> (0:w288:i32)  [unwired: 1 out]
                n176 = property on="Test Ring" class="Ring (strict)"("Value"=w288, "Strings []"=w287) -> ()  [unwired: 2 in, 2 out]
                n177 = property on="Test Ring" class="Ring (strict)"("Visible"=TRUE) -> ()  [unwired: 2 in, 2 out]
                n178 = property on="Test Slider" class="Slide (strict)"("Visible"=FALSE) -> ()  [unwired: 2 in, 2 out]
              }
              frame Default {
                n179 = property on="Test Ring" class="Ring (strict)"("Visible"=FALSE) -> ()  [unwired: 2 in, 2 out]
                n180 = property on="Test Slider" class="Slide (strict)"("Visible"=FALSE) -> ()  [unwired: 2 in, 2 out]
              }
              frame "Brightness  **", "Color Level  **", "Compression  **", "FPS  **", "Sharpness  **" {
                n181 = call <vilib>:"NT Read Number.vi"("Name"=w299) -> ("Numeric"=w298:dbl)  [unwired: 9 in, 1 out]
                n182 = local write "Test Slider"(w298) -> ()
                n183 = property on="Test Ring" class="Ring (strict)"("Visible"=FALSE) -> ()  [unwired: 2 in, 2 out]
                n184 = property on="Test Slider" class="Slide (strict)"("Visible"=TRUE, "Scale.Maximum"=100.0 ("Scale.Range:Maximum")) -> ()  [unwired: 2 in, 2 out]
              }
            }
          }
        }
        n185 = property on="Progress" class="Clust (strict)"("Visible"=FALSE) -> ()  [unwired: 2 in, 2 out]
      }
      event "Test Name": Mouse Enter {
        # "Populate the ring with the list of tests"
        n186 = event-data() -> ()  [unwired: 1 in, 1 out]
        n187 = call <vilib>:"NT Read String Array.vi"("Name"="TestMode/TestList") -> ("String Array"=w307:string[])  [unwired: 9 in, 1 out]
        n188 = Build Array (concatenate)("Select the test to run...", w307) -> (w306:string[])
        n189 = property on="Test Name" class="Ring (strict)"("Strings []"=w306) -> ()  [unwired: 2 in, 2 out]
      }
      event "Test Name": Value Change {
        w309 = FALSE ("Visible")
        # "Tell the robot the test name to run"
        n190 = event-data() -> ("NewVal"=w313:u16)  [unwired: 1 in]
        n191 = property on="Test Name" class="Ring (strict)"() -> ("Strings []"=w314:string[])  [unwired: 2 in, 2 out]
        n192 = local write "Progress"(T10 {"Test Progress"=0, "Test Progress Text"=""} ("Progress")) -> ()
        n193 = Index Array(array=w314, index=w313) -> (element=w312:string)
        n194 = call <vilib>:"NT Write String.vi"("String"=w312, "Name"="TestMode/TestName") -> ()  [unwired: 9 in, 1 out]
        n195 = property on="Progress" class="Clust (strict)"("Visible"=TRUE) -> ()  [unwired: 2 in, 2 out]
        n196 = property on="Motor" class="Clust (strict)"("Visible"=w309) -> ()  [unwired: 2 in, 2 out]
        n197 = property on="Test Slider" class="Slide (strict)"("Visible"=w309) -> ()  [unwired: 2 in, 2 out]
        n198 = property on="On/Off" class="Bool (strict)"("Visible"=w309) -> ()  [unwired: 2 in, 2 out]
        n199 = property on="Rev/Fwd" class="Clust (strict)"("Visible"=w309) -> ()  [unwired: 2 in, 2 out]
        n200 = property on="Test Ring" class="Ring (strict)"("Visible"=w309) -> ()  [unwired: 2 in, 2 out]
      }
      event "Listbox": Double Click {
        n201 = event-data() -> ("PlatMods.Shift"=w317:bool, "Row"=w319:i32)  [unwired: 1 in]
        n202 = case shown="True" w317 {
          tunnel: w319 -> [w323 _]
          tunnel: 1 -> [w322 _]
          frame False {
            n203 = property on="Listbox" class="LstBox (strict)"() -> ("Item Symbols"=w321:i32[])  [unwired: 2 in, 2 out]
            n204 = Replace Array Subset(array=w321, new element=w322, index=w323) -> (w320:i32[])
            n205 = property on="Listbox" class="LstBox (strict)"("Item Symbols"=w320) -> ()  [unwired: 2 in, 2 out]
          }
          frame True {
            w324 = 0 ("Top Row")
            n206 = property on="Listbox" class="LstBox (strict)"() -> ("Number of Rows"=w326:u32)  [unwired: 2 in, 2 out]
            n207 = Initialize Array(0, w326) -> (w325:i32[])
            n208 = property on="Listbox" class="LstBox (strict)"("Top Row"=w324, "Value"=w324, "Item Symbols"=w325) -> ()  [unwired: 2 in, 2 out]
          }
        }
      }
      event "Listbox": Key Down {
        n209 = event-data() -> ("VKey"=w330:T18)  [unwired: 1 in]
        n210 = case shown="\"Left\", \"Right\"" w330 {
          selector: w330 -> [w335 _]
          tunnel: eventvkey."Left" ("VKey") -> [w333 _]
          frame "Left", "Right" {
            n211 = Equal?(x=w333, y=w335) -> (x = y?=w334:bool)
            n212 = Select(t=0, s=w334, f=1) -> (s? t:f=w336:i32)
            n213 = property on="Listbox" class="LstBox (strict)"() -> ("Item Symbols"=w339:i32[])  [unwired: 2 in, 2 out]
            n214 = Replace Array Subset(array=w339, new element=w336, index="Listbox") -> (w338:i32[])
            n215 = property on="Listbox" class="LstBox (strict)"("Item Symbols"=w338) -> ()  [unwired: 2 in, 2 out]
          }
          frame Default {
          }
        }
      }
      event "DB Camera Config": Value Change {
        n216 = event-data() -> ("NewVal"=w343:bool)  [unwired: 1 in]
        n217 = case shown="False" w343 {
          tunnel: w342 -> [w352 _]
          tunnel: [w345 w363] -> w341
          tunnel: w340 -> [w344 w363]
          frame False {
            w359 = "Camera"
            w362 = FALSE ("Visible")
            n218 = local read "Camera Settings"() -> (w351:T2)
            n219 = Index Array(array=w352) -> (element=w355:cluster{string[]})  [unwired: 1 in]
            n220 = Unbundle(w351) -> ("Frame Rate"=w350:i32, "Compression"=w349:i32, "Size"=w353:u16)
            n221 = Unbundle(w355) -> (w354:string[])
            n222 = Index Array(array=w354, index=w353) -> (element=w348:string)
            n223 = call-poly <vilib>:"Write Key.vi"("section"=w359, "value"=w348, "key"="Size", "refnum"=w344) -> ("refnum out"=w361:T17)  [unwired: 2 in, 5 out]
            n224 = call-poly <vilib>:"Write Key.vi"("section"=w359, "value"=w350, "key"="FrameRate", "refnum"=w361) -> ("refnum out"=w360:T17)  [unwired: 1 in, 6 out]
            n225 = property on="Camera Settings" class="Clust (strict)"("Visible"=w362) -> ()  [unwired: 2 in, 2 out]
            n226 = local write "DB Camera Config"(w362) -> ()
            n227 = call-poly <vilib>:"Write Key.vi"("section"=w359, "value"=w349, "key"="Compression", "refnum"=w360) -> ("refnum out"=w346:T17)  [unwired: 1 in, 6 out]
            n228 = call <vilib>:"Close Config Data.vi"("refnum"=w346) -> ("file path"=w347:path)  [unwired: 2 in, 8 out]
            n229 = call <vilib>:"Open Config Data.vi"("configuration file path"=w347) -> ("refnum"=w345:T17)  [unwired: 8 in, 2 out]
          }
          frame True {
            n230 = property on="Camera Settings" class="Clust (strict)"("Visible"=TRUE) -> ()  [unwired: 2 in, 2 out]
          }
        }
      }
      event "Camera Settings": Value Change {
        n231 = event-data() -> ("NewVal"=w376:T2)  [unwired: 1 in]
        n232 = Index Array(array=w372) -> (element=w371:cluster{string[]})  [unwired: 1 in]
        n233 = Unbundle(w376) -> ("Frame Rate"=w367:i32, "Compression"=w366:i32, "Size"=w369:u16)
        n234 = Unbundle(w371) -> (w370:string[])
        n235 = Index Array(array=w370, index=w369) -> (element=w368:string)
        n236 = Format Into String(format string="%s   %dfps   %d%%", w368, w367, w366) -> (resulting string=w373:string)  [unwired: 2 in, 1 out]
        n237 = Build Array(w373) -> (w374:string[])
        n238 = property on="DB Camera Config" class="Bool (strict)"("Strings [4]"=w374) -> ()  [unwired: 2 in, 2 out]
      }
      event "Motor.Enable": Value Change {
        n239 = event-data() -> ("NewVal"=w382:bool)  [unwired: 1 in]
        n240 = Unbundle("Motor") -> ("Value"=w381:dbl)  [unwired: 1 out]
        n241 = Select(t=w381, s=w382, f=0.0) -> (s? t:f=w379:dbl)
        n242 = call <vilib>:"NT Write Number.vi"("Numeric"=w379, "Name"=w378) -> ()  [unwired: 9 in, 1 out]
      }
      event "Test Slider": Value Change {
        n243 = event-data() -> ("NewVal"=w385:dbl)  [unwired: 1 in]
        n244 = call <vilib>:"NT Write Number.vi"("Numeric"=w385, "Name"=w386) -> ()  [unwired: 9 in, 1 out]
      }
      event "On/Off": Value Change {
        n245 = event-data() -> ("NewVal"=w390:bool)  [unwired: 1 in]
        n246 = Boolean To (0,1)(Boolean=w390) -> (0, 1=w389:i16)
        n247 = call <vilib>:"NT Write Number.vi"("Numeric"=w389, "Name"=w388) -> ()  [unwired: 9 in, 1 out]
      }
      event "Rev/Fwd": Value Change {
        n248 = event-data() -> ("NewVal.Forward"=w398:bool, "NewVal.Reverse"=w397:bool)  [unwired: 1 in]
        n249 = Boolean To (0,1)(Boolean=w398) -> (0, 1=w394:i16)
        n250 = Boolean To (0,1)(Boolean=w397) -> (0, 1=w396:i16)
        n251 = Negate(x=w396) -> (-x=w395:i16)
        n252 = Add(x=w394, y=w395) -> (x+y=w393:i16)
        n253 = call <vilib>:"NT Write Number.vi"("Numeric"=w393, "Name"=w392) -> ()  [unwired: 9 in, 1 out]
      }
      event "Test Ring": Value Change {
        n254 = event-data() -> ("NewVal"=w402:u16)  [unwired: 1 in]
        n255 = property on="Test Ring" class="Ring (strict)"() -> ("Strings []"=w403:string[])  [unwired: 2 in, 2 out]
        n256 = Index Array(array=w403, index=w402) -> (element=w401:string)
        n257 = call <vilib>:"NT Write String.vi"("String"=w401, "Name"=w400) -> ()  [unwired: 9 in, 1 out]
      }
      event "Rec Mode": Value Change {
        # "Update globals for recording mode and path to read log from.\nClear when logging and let NetworkTables set path for vision to\nuse."
        n258 = event-data() -> ("NewVal"=w413:enum32{"Stop", "Record", "Playback"})  [unwired: 1 in]
        n259 = case shown="\"Stop\", \"Record\"" w413 {
          tunnel: w412 -> [_ w415 w423]
          tunnel: [_ _ w422] -> w409
          tunnel: [_ _ w421] -> _
          tunnel: w407 -> [_ _ w419]
          tunnel: cluster{i32, i32} {-250, 170} -> [_ _ w418]
          tunnel: [_ _ T19 {"Image Size"=TRUE, "Image Type"=TRUE, "Pixel Value"=TRUE, "ROI Information"=TRUE, "Zoom Factor"=FALSE} ("Image Information Shown:All Elements")] -> w405
          tunnel: [_ _ TRUE ("Zoom Factor")] -> w404
          frame Default {
          }
          frame "Stop", "Record" {
            # "Place Window too"
            n260 = invoke class="VI" method="FP.Close"(reference=w415) -> (reference out=w414:refnum<vi>)  [unwired: 2 in, 2 out]
            n261 = invoke class="VI" method="Abort VI"(reference=w414) -> ()  [unwired: 2 in, 3 out]
          }
          frame "Playback" {
            n262 = call "Open Playback Panel.vi"("Offset"=w418, "DB VI Ref"=w419, "Playback in"=w423) -> ("Playback out"=w420:refnum<vi>)  [unwired: 8 in]
            n263 = register-events(w420) -> (reference out=w422:refnum<event-registration>, error out=w421:errorcluster)  [unwired: 2 in]
          }
        }
        n264 = global write "WPI_DashboardLogging Global.vi" "Recording"(w413) -> ()
        n265 = global write "WPI_DashboardLogging Global.vi" "Logging Filename"(path "") -> ()
        n266 = property on="Camera Image" class="ImageControl"("Image Information Shown"=w405, "Image Information Visible"=w404) -> ()  [unwired: 2 in, 2 out]
        n267 = call <vilib>:"WPI_DashboardNT Log FieldName Cache.vi"("Operation"=enum16{"Lookup/Add", "Index", "Clear"}."Clear") -> ()  [unwired: 8 in, 3 out]
      }
      event Panel Close {
        w424 = enum32{"Stop", "Record", "Playback"}."Stop" ("Rec Mode")
        n268 = event-data() -> ()  [unwired: 1 in, 4 out]
        n269 = local write "Rec Mode"(w424) -> ()
        n270 = global write "WPI_DashboardLogging Global.vi" "Recording"(w424) -> ()
      }
      event Panel Close {
        # "Abort playback window and ourself"
        n271 = event-data() -> ()  [unwired: 1 in, 4 out]
        n272 = invoke class="VI" method="FP.Close"(reference=w429) -> (reference out=w428:refnum<vi>)  [unwired: 2 in, 2 out]
        n273 = invoke class="VI" method="Abort VI"(reference=w428) -> (error out=w427:errorcluster)  [unwired: 2 in, 2 out]
        n274 = invoke class="VI" method="Abort VI"(error in=w427) -> ()  [unwired: 2 in, 3 out]
      }
    }
  }
  n275 = property on="On/Off" class="Bool (strict)"("Visible"=w25) -> ()  [unwired: 2 in, 2 out]
  n276 = property on="Motor" class="Clust (strict)"("Visible"=w25) -> ()  [unwired: 2 in, 2 out]
  n277 = property on="Progress" class="Clust (strict)"("Visible"=w25) -> ()  [unwired: 2 in, 2 out]
  n278 = property on="Test Ring" class="Ring (strict)"("Visible"=w25) -> ()  [unwired: 2 in, 2 out]
  n279 = property on="Rev/Fwd" class="Clust (strict)"("Visible"=w25) -> ()  [unwired: 2 in, 2 out]
  n280 = property on="Camera Settings" class="Clust (strict)"("Visible"=w25) -> ()  [unwired: 2 in, 2 out]
  n281 = local write "DB Camera Config"(w25) -> ()
  n282 = global write "WPI_DashboardLogging Global.vi" "Recording"(w8) -> ()
  n283 = local write "Rec Mode"(w8) -> ()
